vi "Read.vi"(8 "error in (no error)":errorcluster, 11 "Boolean in":refnum<class "UI-Bus_Variant.lvclass">) -> (0 "error out":errorcluster, 2 "Variant":variant, 3 "Boolean out":refnum<class "UI-Bus_Variant.lvclass">)   [LabVIEW 2021, in "UI-Bus_Variant.lvclass"]
doc: "Abstract Data Classes 2.1.1.13\nTim Streeter - TSA\nCopyright (c) 2025, TSA"
uses:
  UI-Bus_Variant.lvclass
  UI-Bus_Variant.lvclass/UI-Bus_Variant.ctl
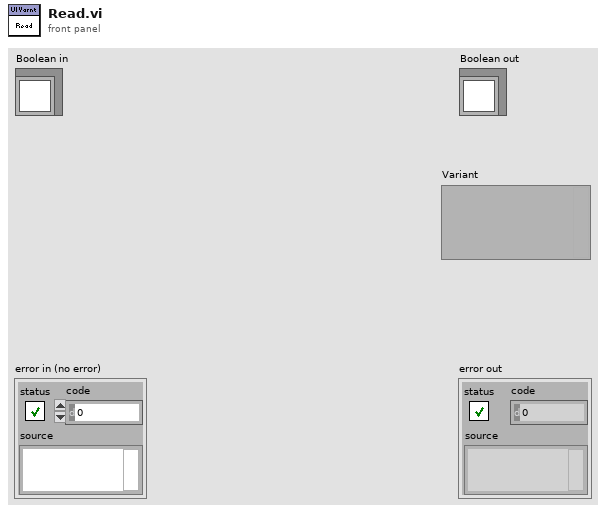
[diagram p1: front panel]
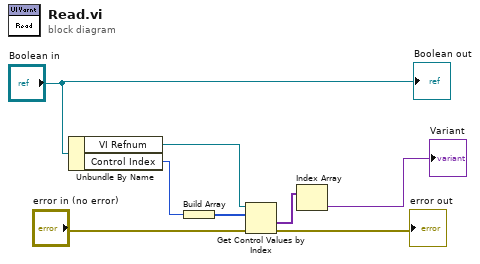
[diagram p0: block diagram]
diagram:
  n1 = Unbundle By Name("Boolean in") -> ("VI Refnum"=w6:refnum<vi>, "Control Index"=w5:i32)
  n2 = Build Array(w5) -> (w4:i32[])
  n3 = Get Control Values by Index(0:w6, 1:w4, 3:"error in (no error)") -> (10:w3:variant[], 11:→"error out":errorcluster)
  n4 = Index Array(array=w3) -> (element=→"Variant":variant)  [unwired: 1 in]
  "Boolean out" <- "Boolean in"
